vi "query unit settings.vi"(8 "error in (no error)":errorcluster, 11 "VISA session":refnum<visa-resource-name>) -> (0 "error out":errorcluster, 2 "Unit Settings":i32, 3 "dup VISA session":refnum<visa-resource-name>)   [LabVIEW 2017]
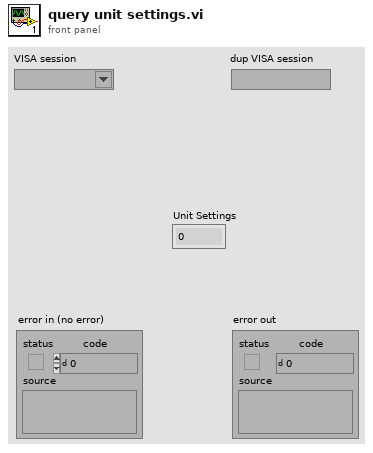
[diagram p1: front panel]
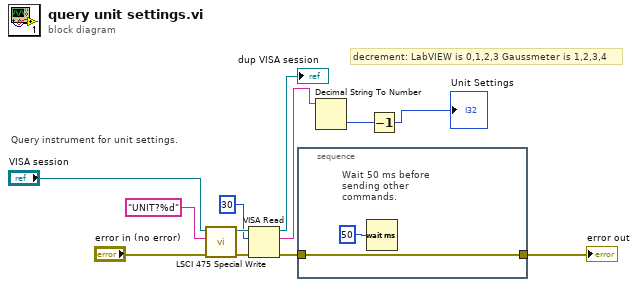
[diagram p0: block diagram]
diagram:
  # "decrement: LabVIEW is 0,1,2,3 Gaussmeter is 1,2,3,4"
  # "Query instrument for unit settings."
  n1 = call "LSCI 475 Special Write.vi"("error in (no error)"="error in (no error)", "Write Buffer (\"\")"="UNIT?%d", "VISA session"="VISA session") -> ("error out"=w8:errorcluster, "dup VISA session"=w9:refnum<visa-resource-name>)  [unwired: 6 in, 1 out]
  n2 = VISA Read(VISA resource name=w9, byte count=u32 30, error in (no error)=w8) -> (VISA resource name out=→"dup VISA session":refnum<visa-resource-name>, read buffer=w3:string, error out=w5:errorcluster)  [unwired: 1 out]
  n3 = stacked-sequence {
    tunnel: w5 -> [w13]
    tunnel: [w13] -> w4
    frame #0 {
      # "Wait 50 ms before\nsending other\ncommands."
      n4 = Wait (ms)(milliseconds to wait=u32 50) -> ()  [unwired: 1 out]
    }
  }
  "error out" <- w4
  n5 = Decimal String To Number(string=w3) -> (number=w2:i32)  [unwired: 2 in, 1 out]
  n6 = Decrement(x=w2) -> (x-1=→"Unit Settings":i32)
